vi "Encode (Structured Append).vi"(8 "error in (no error)":errorcluster, 10 "Data":string, 11 "QR Code Encoder in":refnum<class "QR Code Encoder.lvclass">) -> (0 "error out":errorcluster, 2 "QR Codes":cluster{"Image Data":u8[][]}[](array[cluster]), 3 "QR Code Encoder":refnum<class "QR Code Encoder.lvclass">)   [LabVIEW 2020, in "feature_detection.lvlib" / "QR Code Encoder.lvclass"]
doc: "Encode the supplied Data into QR Code Image Data."
uses:
  QR Code Encoder.lvclass
  QR Code Encoder.lvclass/QR Code Encoder.ctl
  common/common.lvlib
  common/bin/gartoolkit_fd_32-1.dll
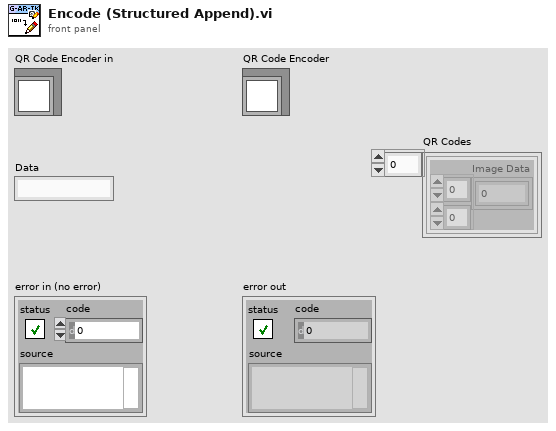
[diagram p1: front panel]
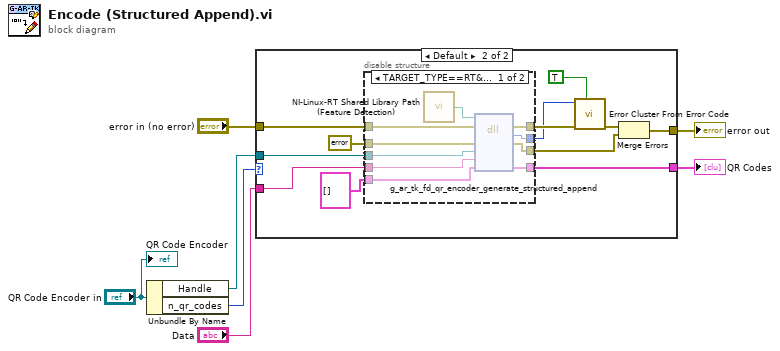
[diagram p0: block diagram]
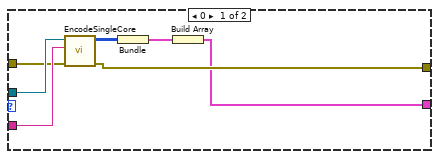
[diagram p2: hidden frame]
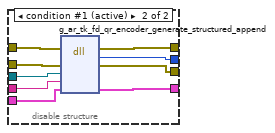
[diagram p3: hidden frame]
diagram:
  n1 = Unbundle By Name("QR Code Encoder in") -> ("Handle"=w6:refnum<data-value>, "n_qr_codes"=w1:u8)
  n2 = case shown="Default" w1 {
    tunnel: w6 -> [w14 w21]
    tunnel: "Data" -> [w13 w20]
    tunnel: "error in (no error)" -> [w12 w19]
    tunnel: [w11 w18] -> w3
    tunnel: [w8 w16] -> w2
    frame 0 {
      n3 = call "EncodeSingleCore.vi"("error in (no error)"=w12, "Data"=w13, "Data Value Reference in"=w14) -> ("error out"=w11:errorcluster, "QR Code Image Data"=w10:u8[][])  [unwired: 7 in]
      n4 = Bundle("QR Code Image Data"=w10) -> (w9:cluster{"QR Code Image Data":u8[][]})  [unwired: 1 in]
      n5 = Build Array(w9) -> (w8:cluster{"QR Code Image Data":u8[][]}[])
    }
    frame Default {
      n6 = disable-structure "Conditional Disable Structure" shown="TARGET_TYPE==RT&&OS==Linux" {
        disable-tunnel: w19 -> [w36 w45]
        disable-tunnel: errorcluster {"status"=FALSE, "code"=0, "source"=""} ("error constant") -> [w32 w44]
        disable-tunnel: [w35 w43] -> w24
        disable-tunnel: [w34 w42] -> w23
        disable-tunnel: [w31 w41] -> w22
        disable-tunnel: w21 -> [w30 w40]
        disable-tunnel: w20 -> [w29 w39]
        disable-tunnel: cluster{u8[][]}[] [] -> [w27 w38]
        disable-tunnel: [w28 w37] -> w16
        frame condition #0 {
          n7 = call "NI-Linux-RT Shared Library Path (Feature Detection).vi"() -> ("Path"=w33:path)
          n8 = dll-call lib="?" fn="g_ar_tk_fd_qr_encoder_generate_structured_append" ("g_ar_toolkit.*.*:g_ar_tk_capture_context_create")(path in=w33, error in=w36, "error_cluster"=w32, "EDVR"=w30, "string"=w29, "output"=w27) -> (error out=w35:errorcluster, w34:i32, "error_cluster"=w31:errorcluster, "output"=w28:cluster{u8[][]}[])  [unwired: 3 in, 1 out]
        }
        frame condition #1 (active) {
          n9 = dll-call lib="C:/serenial/lib/g-augmented-reality-toolkit/LabVIEW/common/bin/gartoolkit_fd_*-1.*" fn="g_ar_tk_fd_qr_encoder_generate_structured_append" ("g_ar_toolkit.*.*:g_ar_tk_capture_context_create")(error in=w45, "error_cluster"=w44, "EDVR"=w40, "string"=w39, "output"=w38) -> (error out=w43:errorcluster, w42:i32, "error_cluster"=w41:errorcluster, "output"=w37:cluster{u8[][]}[])  [unwired: 4 in, 1 out]
        }
      }
      n10 = call <vilib>:"Error Cluster From Error Code.vi"("show call chain? (False)"=TRUE, "error in (no error)"=w24, "error code (0)"=w23) -> ("error out"=w26:errorcluster)  [unwired: 6 in]
      n11 = Merge Errors(w26, w22) -> (w18:errorcluster)
    }
  }
  "error out" <- w3
  "QR Codes" <- w2
  "QR Code Encoder" <- "QR Code Encoder in"
